vi "Parse Custom Route String.vi"(10 "Destination In":string, 11 "Source In":string) -> (0 "Module?":bool, 1 "Module Out":string, 2 "Destination Out":string, 3 "Source Out":string)   [LabVIEW 2020, in "NI Synchronization Engine.lvlib"]
uses:
  NI Synchronization Engine.lvlib
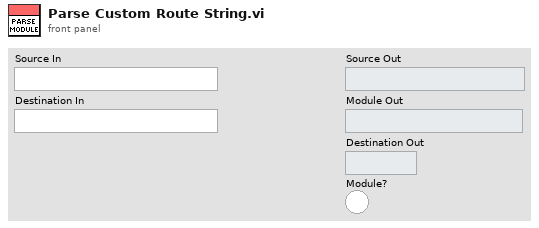
[diagram p1: front panel]
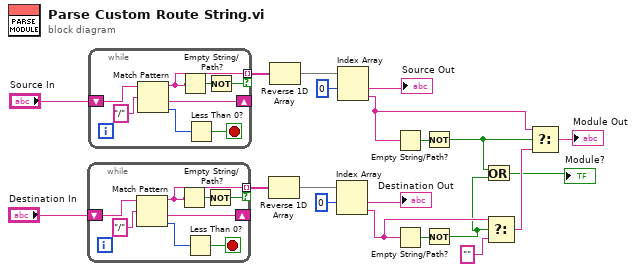
[diagram p0: block diagram]
diagram:
  n1 = while {
    shift-right: [w24] -> _
    shift-left: "Destination In" -> [w28]
    tunnel: [w22] -> w12 mode=indexing if=w21
    stop <- w25 stop-if-true
    n2 = Match Pattern(string=w28, regular expression="/") -> (before substring=w22:string, after substring=w24:string, offset past match=w26:i32)  [unwired: 1 in, 1 out]
    n3 = Empty String/Path?(string/path=w22) -> (empty?=w23:bool)
    n4 = Less Than 0?(x=w26) -> (x < 0?=w25:bool)
    n5 = Not(x=w23) -> (.not. x?=w21:bool)
  }
  n6 = while {
    shift-right: [w32] -> _
    shift-left: "Source In" -> [w36]
    tunnel: [w30] -> w19 mode=indexing if=w29
    stop <- w33 stop-if-true
    n7 = Match Pattern(string=w36, regular expression="/") -> (before substring=w30:string, after substring=w32:string, offset past match=w34:i32)  [unwired: 1 in, 1 out]
    n8 = Empty String/Path?(string/path=w30) -> (empty?=w31:bool)
    n9 = Less Than 0?(x=w34) -> (x < 0?=w33:bool)
    n10 = Not(x=w31) -> (.not. x?=w29:bool)
  }
  n11 = Reverse 1D Array(array=w12) -> (reversed array=w14:string[])
  n12 = Reverse 1D Array(array=w19) -> (reversed array=w17:string[])
  n13 = Index Array(array=w14, index #1=0 ("index")) -> (element #1=→"Destination Out":string, element #2=w6:string)  [unwired: 1 in]
  n14 = Index Array(array=w17, index #1=0 ("index")) -> (element #1=→"Source Out":string, element #2=w5:string)  [unwired: 1 in]
  n15 = Empty String/Path?(string/path=w5) -> (empty?=w15:bool)
  n16 = Empty String/Path?(string/path=w6) -> (empty?=w7:bool)
  n17 = Not(x=w15) -> (.not. x?=w3:bool)
  n18 = Not(x=w7) -> (.not. x?=w2:bool)
  n19 = Or(x=w3, y=w2) -> (x .or. y?=→"Module?":bool)
  n20 = Select(t=w6, s=w2, f="") -> (s? t:f=w8:string)
  n21 = Select(t=w5, s=w3, f=w8) -> (s? t:f=→"Module Out":string)
